vi "Build Tree From Cluster.vi"(7 "Action":T3, 8 "error in":errorcluster, 10 "Display Items":T2(array[cluster]), 11 "Tree Ref":refnum<vi>) -> (0 "error out":errorcluster, 3 "Tree Ref Out":refnum<vi>)   [LabVIEW 2023]
doc: "Take a cluster reference and build a tree of all items in cluster. Set tags of items as \"[row number] item name\" so all tags are unique. Set glyph of its to indicate data type. Set selection color to gray and font size to 18pt."
uses:
  controls/action enum.ctl
panel:
  out "Tree Item Array":T1(array[cluster])
  in  "Tree":string[](tree)
  in  "C1":T4
  # "Debug Cluster"
  # "if display items empty, use this cluster for debug:"
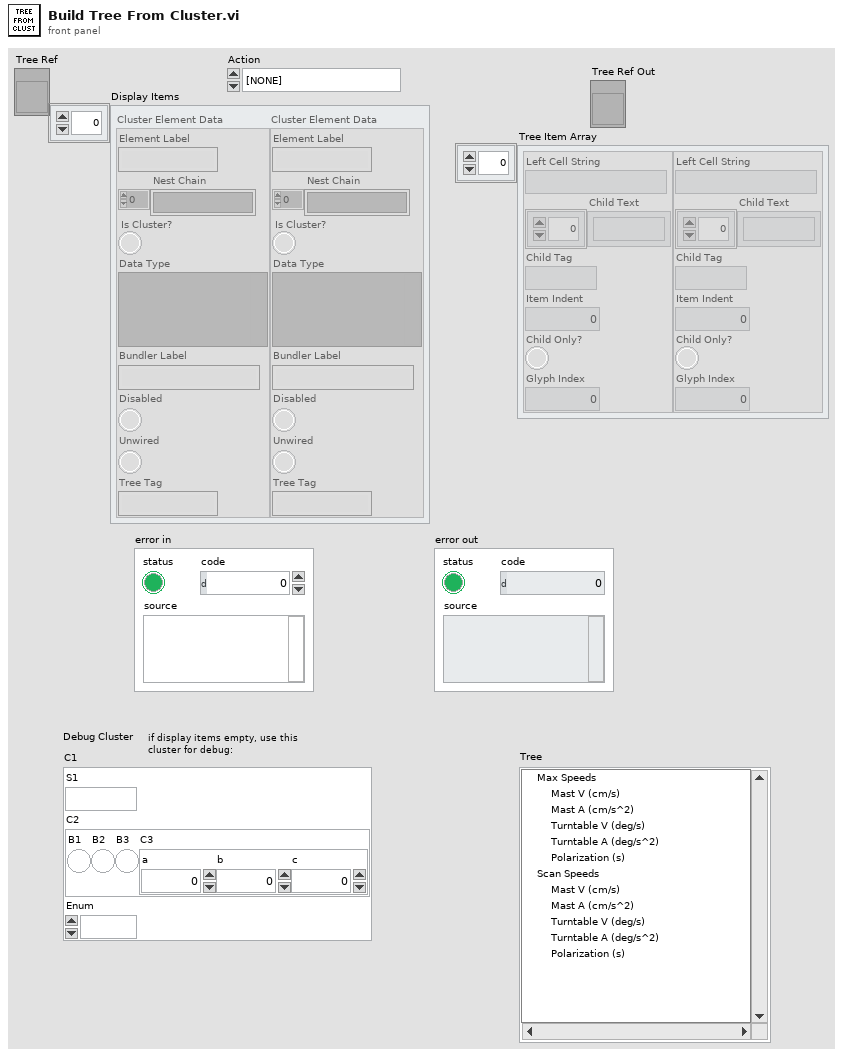
[diagram p1: front panel]
types:
  T1 = cluster{"Left Cell String":string, "Child Text":string[], "Child Tag":string, "Item Indent":i32, "Child Only?":bool, "Glyph Index":i32}[]
  T2 = cluster{"Element Label":string, "Nest Chain":string[], "Is Cluster?":bool, "Data Type":variant, "Bundler Label":string, "Disabled":bool, "Unwired":bool, "Tree Tag":string}[]
  T3 = typedef "action enum.ctl" = enum16{"[NONE]", "APP_SEPARATOR", "Wire Bundle", "Wire Unbundle", "Terminal Unbundle", "Terminal Bundle", "Bundler Move Up", "Bundler Move Down", "Bundler Insert", "Bundler Remove", "Bundler Remove Unwired", "Bundler Reorder", "In Place Insert", "In Place Remove", "In Place Remove Unwired", "In Place Reorder", "Wire Properties", "Wire Method", "Terminal Properties", "Terminal Method", "Property Move Up", "Property Move Down", "Properties Insert", "Properties Remove", "Properties Remove Unwired", "Properties Reorder", "Method Change", "Class For Constant", "Class For Control", "Class For Node", "Class Name to Clipboard"}
  T4 = cluster{"S1":string, "C2":cluster{"B1":bool, "B2":bool, "B3":bool, "C3":cluster{"a":dbl, "b":i32, "c":u8}}, "Enum":enum16{""}}
  T5 = cluster{"image type":i32, "image depth":i32, "image":u8[], "mask":u8[], "colors":u32[], "Rectangle":cluster{"left":i16, "top":i16, "right":i16, "bottom":i16}}
  T6 = typedef "Cluster Element Description.ctl" = cluster{"Element Label":string, "Nest Chain":string[], "Is Cluster?":bool, "Data Type":variant, "Bundler Label":string, "Disabled":bool, "Unwired":bool, "Tree Tag":string}
  T7 = cluster{"left":i16, "top":i16, "right":i16, "bottom":i16}
  T8 = typedef "imagedata.ctl" = cluster{"image type":i32, "image depth":i32, "image":u8[], "mask":u8[], "colors":u32[], "Rectangle":cluster{"left":i16, "top":i16, "right":i16, "bottom":i16}}
  T9 = cluster{"Left Cell String":string, "Child Text":string[], "Child Tag":string, "Item Indent":i32, "Child Only?":bool, "Glyph Index":i32}
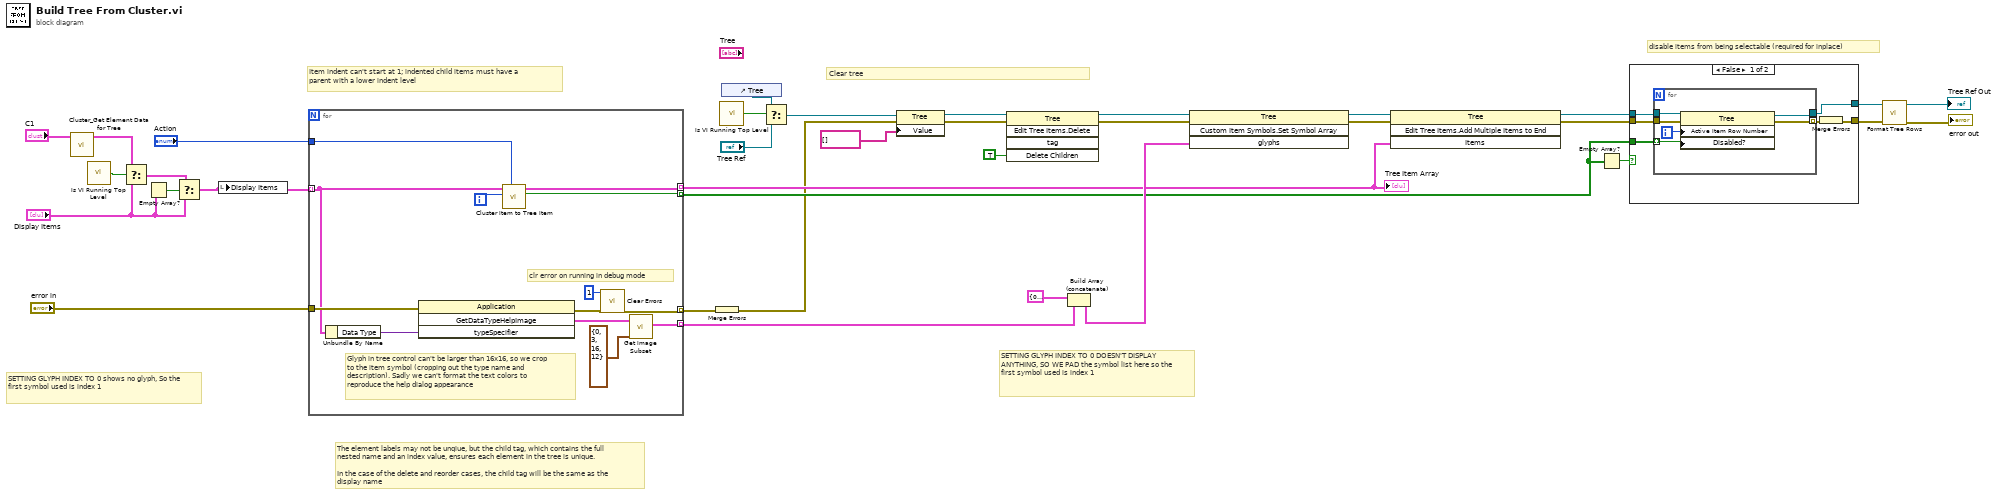
[diagram p0: block diagram]
diagram:
  # "Item indent can't start at 1; indented child items must have a parent with a lower indent level"
  # "Clear tree"
  # "SETTING GLYPH INDEX TO 0 shows no glyph, So the first symbol used is index 1"
  # "disable items from being selectable (required for inplace)"
  # "The element labels may not be unqiue, but the child tag, which contains the full nested name and an index value, ensures each element in the tree is unique. \n\nIn the case of the delete and reorder cases, the child tag will be the same as the display name"
  # "SETTING GLYPH INDEX TO 0 DOESN'T DISPLAY ANYTHING, SO WE PAD the symbol list here so the first symbol used is index 1"
  n1 = call "Cluster_Get Element Data for Tree.vi"("Data Type"="C1") -> ("Cluster Element Data Aray"=w7:T6[])  [unwired: 10 in]
  n2 = call "Is VI Running Top Level.vi"() -> ("Top Level?"=w21:bool)  [unwired: 5 in]
  n3 = Select(t=w7, s=w21, f="Display Items") -> (s? t:f=w20:T6[])
  n4 = Empty Array?(array="Display Items") -> (empty?=w19:bool)
  n5 = Select(t=w20, s=w19, f="Display Items") -> (s? t:f=w5:T6[])
  n6 = local write "Display Items"(w5) -> ()
  n7 = for {
    tunnel: w5 -> [w37] mode=indexing
    tunnel: [w40] -> w18 mode=indexing
    tunnel: [w46] -> w32 mode=indexing
    tunnel: "Action" -> [w38]
    tunnel: "error in" -> [w44]
    tunnel: [w42] -> w15 mode=indexing
    tunnel: [w39] -> w9 mode=indexing
    i -> [w36]
    # "clr error on running in debug mode"
    # "Glyph in tree control can't be larger than 16x16, so we crop to the item symbol (cropping out the type name and description). Sadly we can't format the text colors to reproduce the help dialog appearance"
    n8 = Unbundle By Name(w37) -> ("Data Type"=w48:variant)
    n9 = invoke class="Application" method="GetDataTypeHelpImage"(error in=w44, "typeSpecifier"=w48) -> (error out=w43:errorcluster, "GetDataTypeHelpImage"=w47:T8)  [unwired: 2 in, 2 out]
    n10 = call "Cluster Item to Tree Item.vi"("Action"=w38, "Index"=w36, "Cluster Element Data"=w37) -> ("Disable"=w39:bool, "Item"=w40:T9)  [unwired: 7 in]
    n11 = call <vilib>:"Clear Errors.vi"("error in (no error)"=w43, "specific error code to clear (0: all)"=1) -> ("error out"=w42:errorcluster)  [unwired: 4 in, 1 out]
    n12 = call <vilib>:"Get Image Subset.vi"("subset rect"=T7 {"left"=0, "top"=3, "right"=16, "bottom"=12}, "image data"=w47) -> ("image subset"=w46:T8)  [unwired: 4 in, 1 out]
  }
  "Tree Item Array" <- w18
  n13 = Merge Errors(w15) -> (w3:errorcluster)
  n14 = call "Is VI Running Top Level.vi"() -> ("Top Level?"=w30:bool)  [unwired: 5 in]
  n15 = control-ref of="Tree"() -> (w28:refnum<vi>)
  n16 = Select(t=w28, s=w30, f="Tree Ref") -> (s? t:f=w27:refnum<vi>)
  n17 = property class="Tree"(reference=w27, error in=w3, "Value"=string[] []) -> (reference out=w4:refnum<vi>, error out=w2:errorcluster)
  n18 = invoke class="Tree" method="Edit Tree Items.Delete"(reference=w4, error in=w2, "Delete Children"=TRUE ("Delete Children?")) -> (reference out=w25:refnum<vi>, error out=w24:errorcluster)  [unwired: 2 in, 3 out]
  n19 = Build Array (concatenate)(T5 {"image type"=0, "image depth"=0, "image"=[], "mask"=[], "colors"=[], "Rectangle"={"left"=0, "top"=0, "right"=0, "bottom"=0}} ("image subset"), w32) -> (w31:T8[])
  n20 = invoke class="Tree" method="Custom Item Symbols.Set Symbol Array"(reference=w25, error in=w24, "glyphs"=w31) -> (reference out=w34:refnum<vi>, error out=w26:errorcluster)  [unwired: 1 in, 2 out]
  n21 = invoke class="Tree" method="Edit Tree Items.Add Multiple Items to End"(reference=w34, error in=w26, "Items"=w18) -> (reference out=w23:refnum<vi>, error out=w22:errorcluster)  [unwired: 1 in, 2 out]
  n22 = Empty Array?(array=w9) -> (empty?=w11:bool)
  n23 = case shown="False" w11 {
    tunnel: w23 -> [w54 w62]
    tunnel: w22 -> [w53 w61]
    tunnel: w9 -> [w51 _]
    tunnel: [w50 w61] -> w14
    tunnel: [w49 w62] -> w13
    frame False {
      n24 = for {
        tunnel: w51 -> [w56] mode=indexing
        tunnel: w53 -> [w59]
        tunnel: [w57] -> w52 mode=indexing
        tunnel: w54 -> [w60]
        tunnel: [w58] -> w49
        i -> [w55]
        n25 = property class="Tree"(reference=w60, error in=w59, "Active Item Row Number"=w55, "Disabled?"=w56) -> (reference out=w58:refnum<vi>, error out=w57:errorcluster)
      }
      n26 = Merge Errors(w52) -> (w50:errorcluster)
    }
    frame True {
    }
  }
  n27 = call "Format Tree Rows.vi"("error in"=w14, "Tree Ref"=w13) -> ("error out"=→"error out":errorcluster, "Tree Ref out"=→"Tree Ref Out":refnum<vi>)  [unwired: 8 in]
